vi "LED2015 Ctlr Cmds_Test.vi"(0 "VISA session":refnum<visa-resource-name>="COM11", 5 "Intensity":dbl(knob) min=0.0 max=100.0 scale=0.0..100.0, 7 "High Gain":bool, 11 "error in (no error)":errorcluster) -> (4 "VISA session out":refnum<visa-resource-name>, 6 "Bytes at Port":u8, 8 "Response":string, 10 "Bytes Read":u8, 15 "error out":errorcluster)   [LabVIEW 2010]
uses:
  <vilib>/Instr/_visa.llb/VISA Flush IO Buffer Mask.ctl
  <vilib>/Instr/_visa.llb/VISA Configure Serial Port (Instr).vi
panel:
  in  "stop":bool
  out "Write Data (string)":string
  out "3 Byte Command":u8[](array[numeric]) format="%02x"
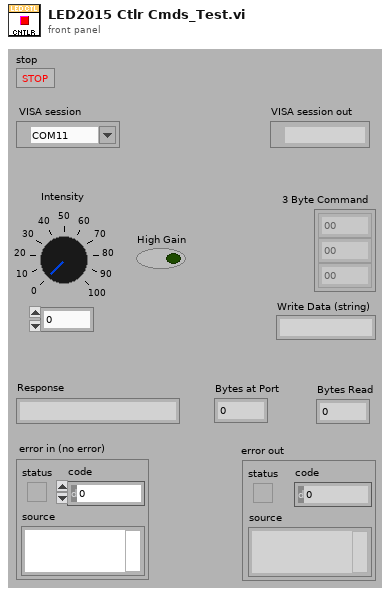
[diagram p1: front panel]
types:
  T1 = typedef "VISA Flush IO Buffer Mask.ctl" = u16
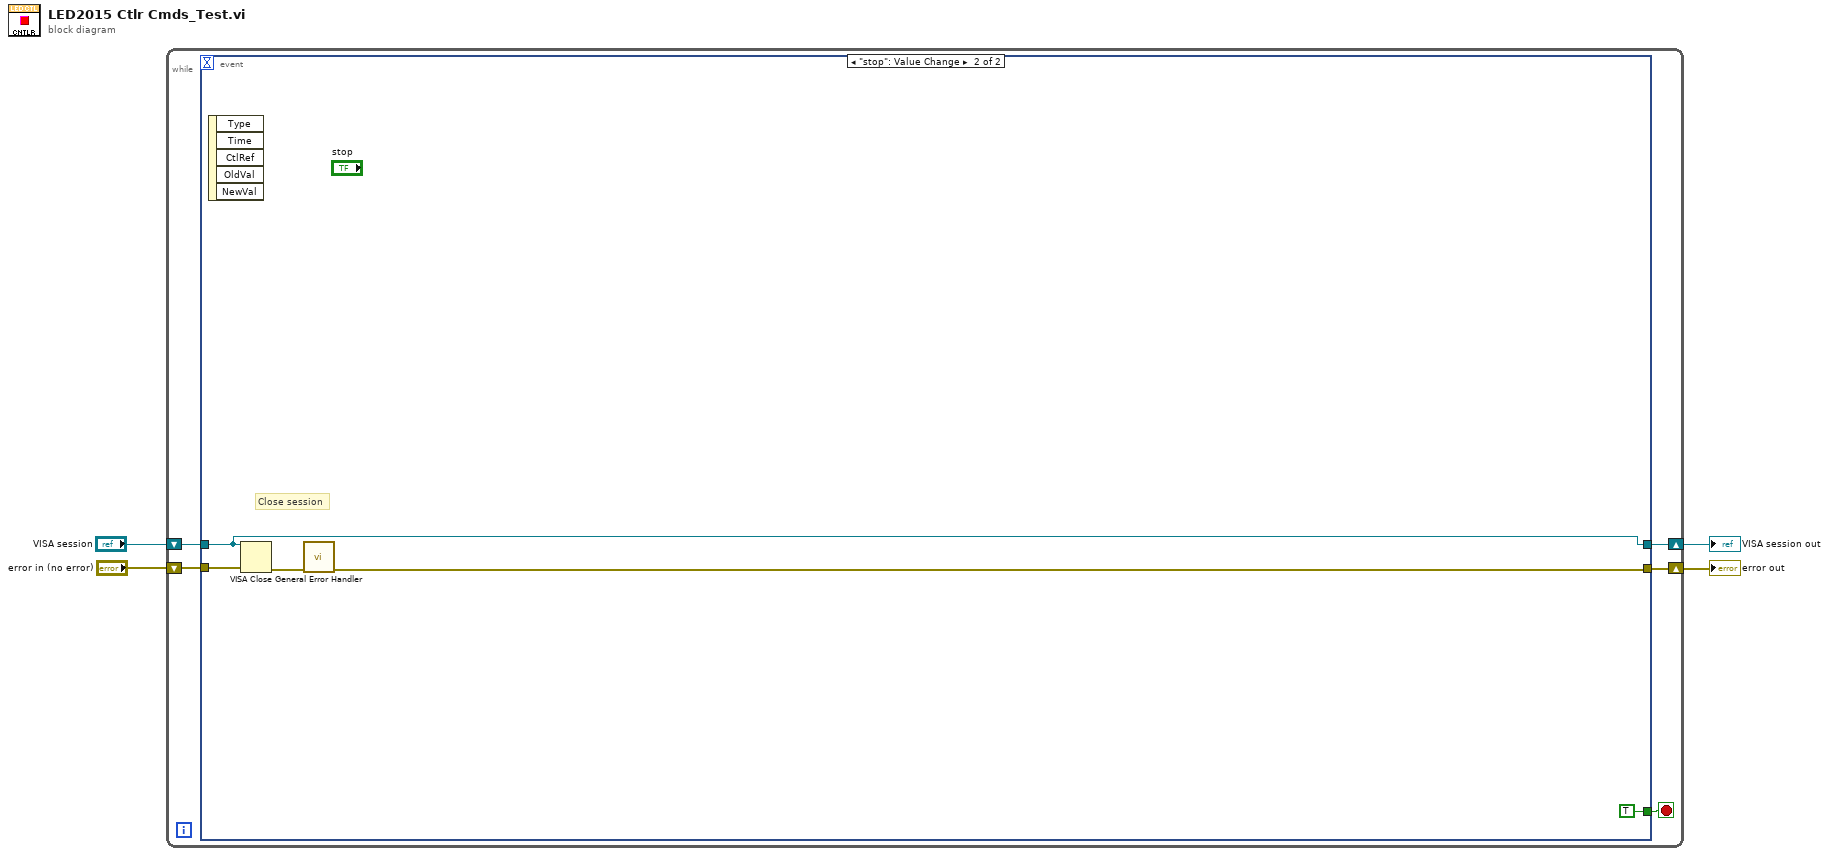
[diagram p0: block diagram]
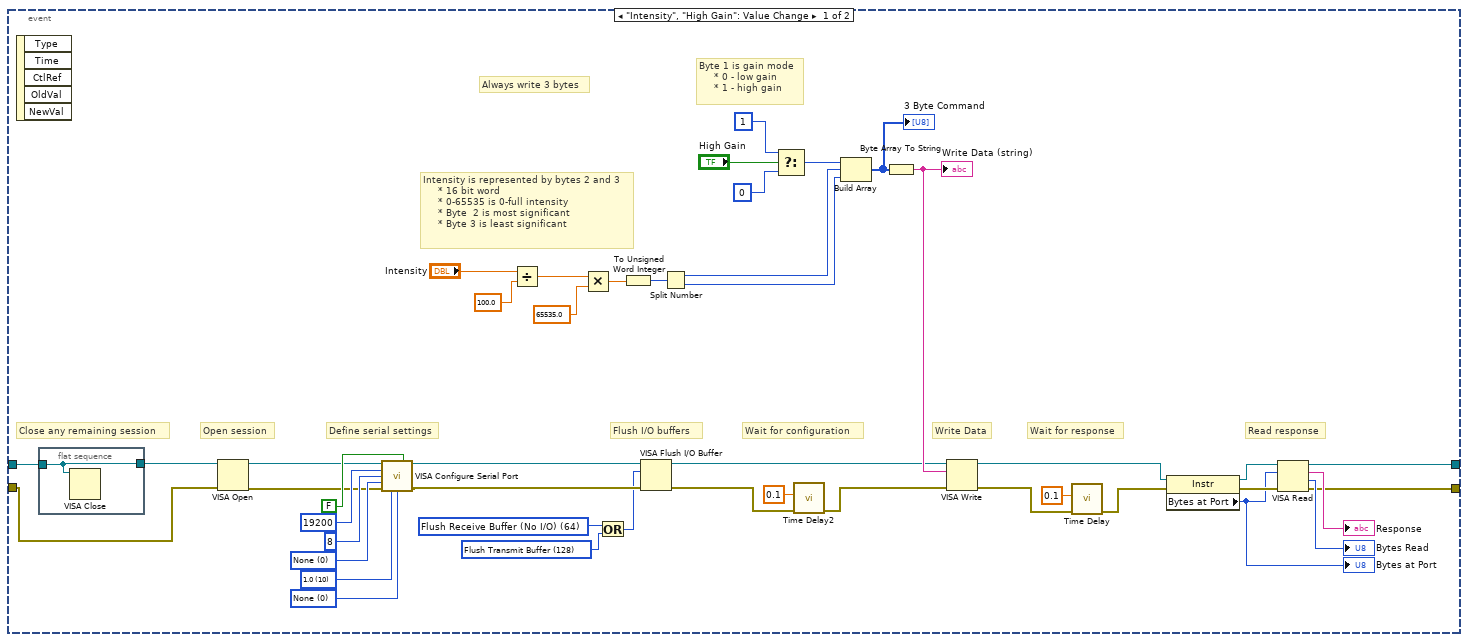
[diagram p2: hidden frame]
diagram:
  n1 = while {
    shift-right: [w6] -> w1
    shift-left: "error in (no error)" -> [w9]
    shift-right: [w7] -> w2
    shift-left: "VISA session" -> [w8]
    stop <- w5 stop-if-true
    n2 = event shown="[1] \"stop\": Value Change" {
      selector: _ -> [_ _]
      dyn-events: _ -> [_ _]
      timeout: _ -> [_ _]
      tunnel: w9 -> [w54 w59]
      tunnel: w8 -> [w53 w57]
      tunnel: [w11 w57] -> w7
      tunnel: [w10 w58] -> w6
      tunnel: [_ TRUE] -> w5
      event "Intensity", "High Gain": Value Change {
        w15 = T1 128 items=["Flush Receive Buffer"=16, "Write Transmit Buffer to Device"=32, "Flush Receive Buffer (No I/O)"=64, "Flush Transmit Buffer"=128] ("y")
        w16 = T1 64 items=["Flush Receive Buffer"=16, "Write Transmit Buffer to Device"=32, "Flush Receive Buffer (No I/O)"=64, "Flush Transmit Buffer"=128] ("Mask")
        w29 = u16 0 items=["None", "XON/XOFF", "RTS/CTS", "XON/XOFF & RTS/CTS", "DTR/DSR", "XON/XOFF & DTR/DSR"] ("Serial Settings:Flow Control")
        w28 = u16 10 items=["1.0"=10, "1.5"=15, "2.0"=20] ("Serial Settings:Stop Bits")
        w27 = u16 0 items=["None", "Odd", "Even", "Mark", "Space"] ("Serial Settings:Parity")
        # "Close any remaining session"
        # "Wait for configuration"
        # "Open session"
        # "Define serial settings"
        # "Flush I/O buffers"
        # "Wait for response"
        # "Read response"
        # "Write Data"
        # "Always write 3 bytes"
        # "Byte 1 is gain mode\n     * 0 - low gain\n     * 1 - high gain"
        # "Intensity is represented by bytes 2 and 3\n     * 16 bit word\n     * 0-65535 is 0-full intensity\n     * Byte  2 is most significant\n     * Byte 3 is least significant"
        n3 = event-data() -> ()  [unwired: 1 in, 5 out]
        n4 = flat-sequence {
          tunnel: [w55] -> w22
          tunnel: w53 -> [w55]
          frame #0 {
            n5 = VISA Close(VISA resource name=w55) -> ()  [unwired: 1 in, 1 out]
          }
        }
        n6 = VISA Open(error in (no error)=w54, VISA resource name=w22) -> (VISA resource name=w23:refnum<visa-resource-name>, error out=w24:errorcluster)  [unwired: 3 in]
        n7 = call-poly "VISA Configure Serial Port"("VISA resource name"=w23, "Enable Termination\nChar (T)"=FALSE ("Message Based Settings:Termination Character Enable"), "baud rate (9600)"=u32 19200 ("Serial Settings:Baud Rate"), "data bits (8)"=u16 8 ("Serial Settings:Data Bits"), "parity (0:none)"=w27, "error in (no error)"=w24, "stop bits (10: 1 bit)"=w28, "flow control (0:none)"=w29) -> ("VISA resource name out"=w17:refnum<visa-resource-name>, "error out"=w21:errorcluster)  [unwired: 6 in]
        n8 = Divide(x="Intensity", y=100.0) -> (x/y=w35:dbl)
        n9 = Multiply(x=w35, y=65535.0) -> (x*y=w36:dbl)
        n10 = Or(x=w16, y=w15) -> (x .or. y?=w14:T1)
        n11 = To Unsigned Word Integer(number=w36) -> (unsigned 16bit integer=w47:u16)
        n12 = VISA Flush I/O Buffer(VISA resource name=w17, mask (16)=w14, error in (no error)=w21) -> (VISA resource name out=w31:refnum<visa-resource-name>, error out=w18:errorcluster)
        n13 = Split Number(x=w47) -> (hi(x)=w34:u8, lo(x)=w13:u8)
        n14 = Select(t=u8 1 ("High Gain"), s="High Gain", f=u8 0 ("Low Gain")) -> (s? t:f=w12:u8)
        n15 = call "Time Delay2"("error in (no error)"=w18, "Delay Time (s)"=0.1) -> ("error out"=w19:errorcluster)  [unwired: 9 in]
        n16 = Build Array(w12, w34, w13) -> (w37:u8[])
        "3 Byte Command" <- w37
        n17 = Byte Array To String(unsigned byte array=w37) -> (string=w32:string)
        "Write Data (string)" <- w32
        n18 = VISA Write(VISA resource name=w31, write buffer=w32, error in (no error)=w19) -> (VISA resource name out=w43:refnum<visa-resource-name>, error out=w45:errorcluster)  [unwired: 1 out]
        n19 = call "Time Delay"("error in (no error)"=w45, "Delay Time (s)"=0.1) -> ("error out"=w44:errorcluster)  [unwired: 9 in]
        n20 = property class="Instr"(reference=w43, error in=w44) -> (reference out=w52:refnum<visa-resource-name>, error out=w51:errorcluster, "Bytes at Port"=w50:u32)
        "Bytes at Port" <- w50
        n21 = VISA Read(VISA resource name=w52, byte count=w50, error in (no error)=w51) -> (VISA resource name out=w11:refnum<visa-resource-name>, read buffer=→"Response":string, return count=→"Bytes Read":u32, error out=w10:errorcluster)
      }
      event "stop": Value Change {
        # "Close session"
        n22 = event-data() -> ()  [unwired: 1 in, 5 out]
        n23 = VISA Close(VISA resource name=w57, error in (no error)=w59) -> (error out=w60:errorcluster)
        n24 = call <vilib>:"General Error Handler.vi"("error in (no error)"=w60) -> ("error out"=w58:errorcluster)  [unwired: 10 in, 4 out]
      }
    }
  }
  "VISA session out" <- w2
  "error out" <- w1
